vi "Set properties.vi"(8 "error in (no error)":errorcluster, 10 "Array of properties":T1[](array[typedef]), 11 "This VI":refnum<vi>) -> (0 "error out":errorcluster)   [LabVIEW 2015, in "ZenGage v3.0 UI.lvclass"]
uses:
  ZenGage v3.0 UI.lvclass
  Type Definitions/General/Set properties.ctl
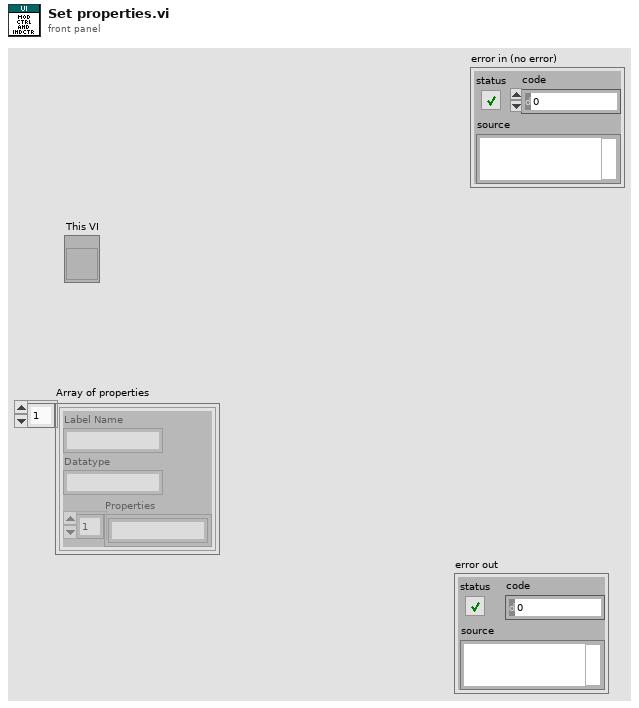
[diagram p1: front panel]
types:
  T1 = typedef "ZenGage v3.0 UI.lvclass/Set properties.ctl" = cluster{"Label Name":string, "Datatype":string, "Properties":string[]}
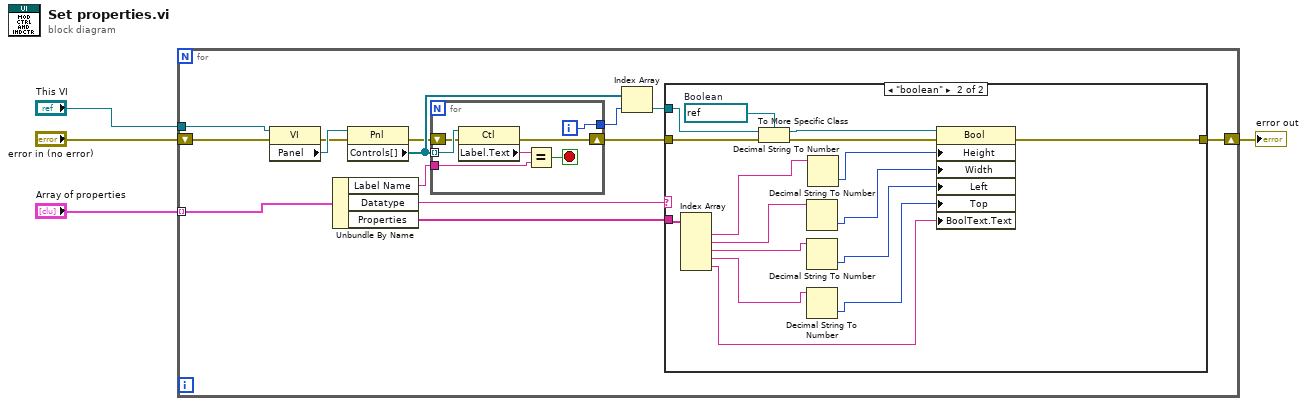
[diagram p0: block diagram]
diagram:
  n1 = for {
    shift-right: [w14] -> w4
    shift-left: "error in (no error)" -> [w11]
    tunnel: "Array of properties" -> [w9] mode=indexing
    tunnel: "This VI" -> [w5]
    n2 = property class="VI"(reference=w5, error in=w11) -> (error out=w12:errorcluster, "Panel"=w15:refnum<vi>)  [unwired: 1 out]
    n3 = Unbundle By Name(w9) -> ("Label Name"=w8:string, "Datatype"=w7:string, "Properties"=w6:string[])
    n4 = property class="Pnl"(reference=w15, error in=w12) -> (error out=w10:errorcluster, "Controls[]"=w13:refnum<vi>[])  [unwired: 1 out]
    n5 = for {
      tunnel: w13 -> [w42] mode=indexing
      tunnel: w8 -> [w40]
      tunnel: [w38] -> w18
      shift-right: [w36] -> w16
      shift-left: w10 -> [w37]
      i -> [w38]
      stop <- w39 stop-if-true
      n6 = property class="Ctl"(reference=w42, error in=w37) -> (error out=w36:errorcluster, "Label.Text"=w41:string)  [unwired: 1 out]
      n7 = Equal?(x=w41, y=w40) -> (x = y?=w39:bool)
    }
    n8 = Index Array(array=w13, index=w18) -> (element=w17:refnum<vi>)
    n9 = case shown="\"boolean\"" w7 {
      tunnel: w17 -> [_ w35]
      tunnel: w16 -> [w19 w32]
      tunnel: [w19 w30] -> w14
      tunnel: w6 -> [_ w29]
      frame "False", Default {
      }
      frame "boolean" {
        w34 = refnum<vi> refnum  # Boolean
        n10 = Index Array(array=w29) -> (element #1=w27:string, element #2=w26:string, element #3=w25:string, element #4=w24:string, element #5=w28:string)  [unwired: 5 in]
        n11 = To More Specific Class(target class=w34, reference=w35, error in=w32) -> (specific class reference=w33:refnum<vi>, error out=w31:errorcluster)
        n12 = Decimal String To Number(string=w26) -> (number=w22:i32)  [unwired: 2 in, 1 out]
        n13 = Decimal String To Number(string=w25) -> (number=w21:i32)  [unwired: 2 in, 1 out]
        n14 = Decimal String To Number(string=w24) -> (number=w20:i32)  [unwired: 2 in, 1 out]
        n15 = Decimal String To Number(string=w27) -> (number=w23:i32)  [unwired: 2 in, 1 out]
        n16 = property class="Bool"(reference=w33, error in=w31, "Height"=w23, "Width"=w22, "Left"=w21, "Top"=w20, "BoolText.Text"=w28) -> (error out=w30:errorcluster)  [unwired: 1 out]
      }
    }
  }
  "error out" <- w4
